vi "Tagged Data to Spreadsheet String.vi"(1 "units":string[](array[string]), 2 "IO in":dbl[](array[numeric]), 3 "channels":string[](array[string])) -> (0 "spreadsheet string":string)   [LabVIEW 2020]
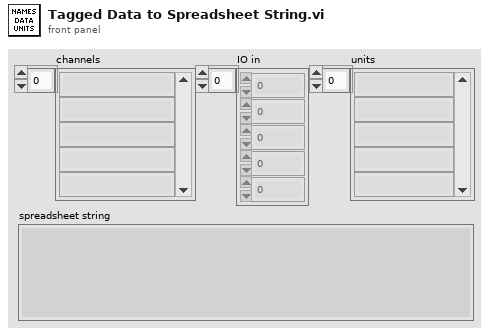
[diagram p1: front panel]
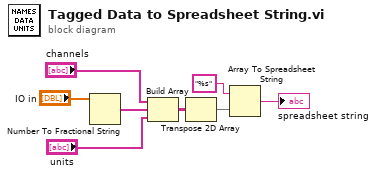
[diagram p0: block diagram]
diagram:
  n1 = Number To Fractional String(number="IO in") -> (F-format string=w4:string[])  [unwired: 3 in]
  n2 = Build Array("channels", w4, "units") -> (w5:string[][])
  n3 = Transpose 2D Array(2D array=w5) -> (transposed array=w7:string[][])
  n4 = Array To Spreadsheet String(array=w7, 3:"%s" ("format string")) -> (spreadsheet string=→"spreadsheet string":string)  [unwired: 1 in]
